vi "Service ID.vi"(8 "error in (no error)":errorcluster, 11 "Service in":refnum<class "Service.lvclass">) -> (0 "error out":errorcluster, 2 "Service ID":string, 3 "Service out":refnum<class "Service.lvclass">)   [LabVIEW 2020, in "HTTP Server.lvlib" / "Service.lvclass"]
uses:
  Service.lvclass
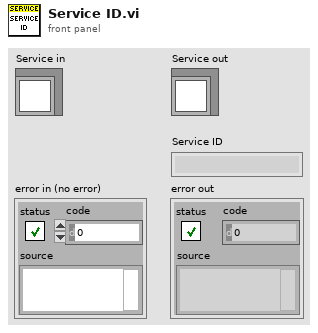
[diagram p1: front panel]
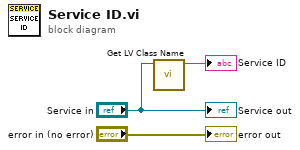
[diagram p0: block diagram]
diagram:
  n1 = call <vilib>:"Get LV Class Name.vi"("object"="Service in") -> ("class name"=→"Service ID":string)  [unwired: 9 in, 1 out]
  "error out" <- "error in (no error)"
  "Service out" <- "Service in"
